vi "CAN.vi"() -> ()   [LabVIEW 2020]
uses:
  Global_Variable/Global.vi
  Global_Variable/A180648.vi
  Libraries/ZLG_CAN/ZLG_CAN.lvlib
panel:
  in  "CAN 通道":u32(ring) items=["0", "1"]
  in  "索引":u32(ring) items=["0", "1", "2", "3", "4", "5", "6", "7", "8"]
  in  "设备类型":u32(ring)=27 items=["PCI5121"=1, "PCI9810"=2, "USBCAN1"=3, "USBCAN2"=4, "PCI9820"=5, "PCI5110"=7, "PC104CAN"=11, "CANETUDP"=12, "PCI9840B"=14, "PC104C2"=15, "PCI9820I"=16, "CANETTCP"=17, "PCIE9221"=24, "PCI5010U"=19, "USBCAN_E_U"=20, "USBCAN_2E_U"=21, "PCI5020U"=22, "PCIE9120I"=27, "PCIE9110I"=28, "PCIE9140I"=29]
  in  "Stop":bool
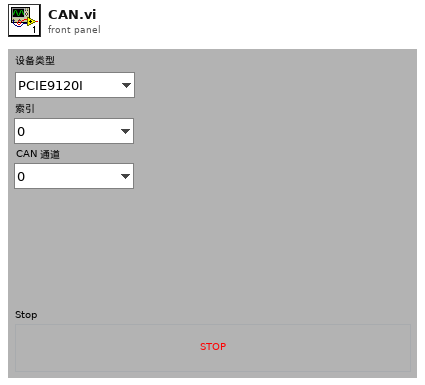
[diagram p1: front panel]
types:
  T1 = cluster{"波特率":u32, "ID":u32, "帧类型":enum8{"标准帧", "扩展帧"}, "帧格式":enum16{"数据帧", "远程帧"}, "周期(ms)":u32}
  T2 = typedef "ZLG_CAN.lvlib/Start_CAN (Reply Payload)--cluster.ctl" = cluster{"Success":bool, "Start_CAN_error":errorcluster}
  T3 = cluster{u8, u8, "y":u8, "y":u8, "y":u8, "y":u8, "y":u8, "y":u8}
  T4 = cluster{"y":u8, "y":u8, "y":u8, u8, u8, "y":u8, "y":u8, "y":u8}
  T5 = cluster{"[0]":u8, "[1]":u8, "[2]":u8, "[3]":u8, "[4]":u8, "[5]":u8, "[6]":u8, "[7]":u8}
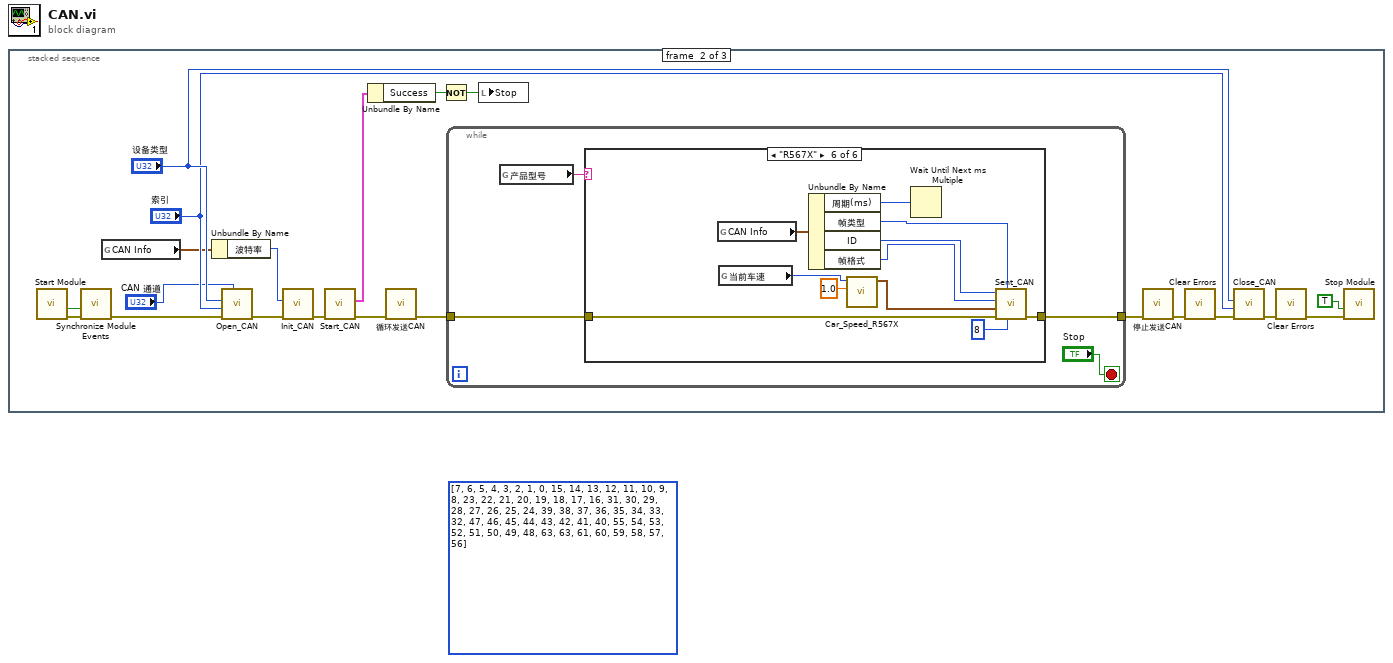
[diagram p0: block diagram]
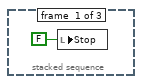
[diagram p2: hidden frame]
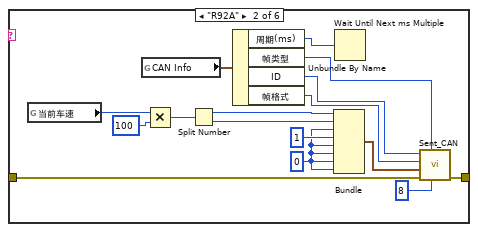
[diagram p4: hidden frame]
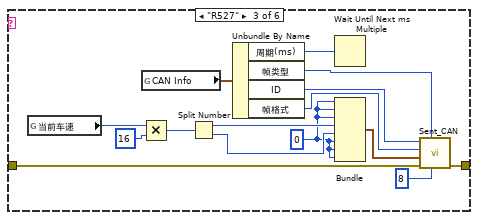
[diagram p5: hidden frame]
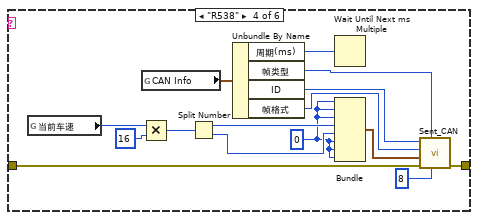
[diagram p6: hidden frame]
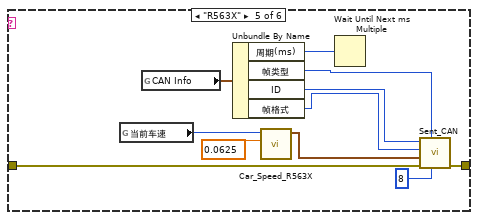
[diagram p7: hidden frame]
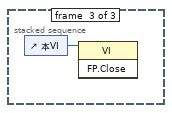
[diagram p8: hidden frame]
diagram:
  (unwired) i32[][] [[7, 6, 5, 4, 3, 2, 1, 0], [15, 14, 13, 12, 11, 10, 9, 8], [23, 22, 21, 20, 19, 18, 17, 16], [31, 30, 29, 28, 27, 26, 25, 24], [39, 38, 37, 36, 35, 34, 33, 32], [47, 46, 45, 44, 43, 42, 41, 40], [55, 54, 53, 52, 51, 50, 49, 48], [63, 63, 61, 60, 59, 58, 57, 56]]
  n1 = stacked-sequence {
    frame #0 {
      n2 = local write "Stop"(FALSE ("Stop")) -> ()
    }
    frame #1 {
      n3 = call "Start Module.vi"() -> ("error out"=w22:errorcluster, "Wait for Event Sync?"=w21:bool)  [unwired: 8 in, 2 out]
      n4 = call "Synchronize Module Events.vi"("error in (no error)"=w22, "Wait for Event Sync?"=w21) -> ("error out"=w20:errorcluster)  [unwired: 9 in]
      n5 = global read "Global.vi" "CAN Info"() -> (w7:T1)
      n6 = Unbundle By Name(w7) -> ("波特率"=w12:u32)
      n7 = call "Open_CAN.vi"("CAN 通道"="CAN 通道", "error in (no error)"=w20, "索引"="索引", "设备类型"="设备类型") -> ("error out"=w17:errorcluster)  [unwired: 7 in]
      n8 = call "Init_CAN.vi"("error in (no error)"=w17, "波特率"=w12) -> ("error out"=w13:errorcluster)  [unwired: 9 in]
      n9 = call "Start_CAN.vi"("error in (no error)"=w13) -> ("error out"=w6:errorcluster, "Reply Payload"=w15:T2)  [unwired: 8 in, 1 out]
      n10 = Unbundle By Name(w15) -> ("Success"=w14:bool)
      n11 = call "循环发送CAN.vi"("错误输入"=w6) -> ("错误输出"=w5:errorcluster)  [unwired: 10 in]
      n12 = Not(x=w14) -> (.not. x?=w2:bool)
      n13 = while {
        tunnel: w5 -> [w26]
        tunnel: [w25] -> w4
        stop <- "Stop" stop-if-true
        n14 = global read "Global.vi" "产品型号"() -> (w23:string)
        n15 = case shown="\"R567X\"" w23 {
          tunnel: w26 -> [w27 w43 w58 w73 w84 w95]
          tunnel: [w27 w42 w57 w72 w83 w94] -> w25
          frame "假", Default {
          }
          frame "R92A" {
            w28 = u8 0 ("y")
            n16 = global read "A180648.vi" "当前车速"() -> (w29:u16)
            n17 = global read "Global.vi" "CAN Info"() -> (w30:T1)
            n18 = Multiply(x=w29, y=u16 100) -> (x*y=w40:u16)
            n19 = Split Number(x=w40) -> (hi(x)=w39:u8, lo(x)=w38:u8)
            n20 = Unbundle By Name(w30) -> ("周期(ms)"=w34:u32, "帧类型"=w32:enum8{"标准帧", "扩展帧"}, "ID"=w31:u32, "帧格式"=w33:enum16{"数据帧", "远程帧"})
            n21 = Bundle(w39, w38, "y"=w28, "y"=u8 1, "y"=w28, "y"=w28, "y"=w28, "y"=w28) -> (w36:T3)  [unwired: 1 in]
            n22 = Wait Until Next ms Multiple(millisecond multiple=w34) -> ()  [unwired: 1 out]
            n23 = call "Sent_CAN.vi"("帧长度"=u8 8, "帧类型"=w32, "error in (no error)"=w43, "帧数据"=w36, "帧格式"=w33, "ID"=w31) -> ("error out"=w42:errorcluster)  [unwired: 5 in]
          }
          frame "R527" {
            w44 = u8 0 ("y")
            n24 = global read "A180648.vi" "当前车速"() -> (w47:u16)
            n25 = Multiply(x=w47, y=u16 16) -> (x*y=w55:u16)
            n26 = global read "Global.vi" "CAN Info"() -> (w48:T1)
            n27 = Split Number(x=w55) -> (hi(x)=w46:u8, lo(x)=w45:u8)
            n28 = Unbundle By Name(w48) -> ("周期(ms)"=w52:u32, "帧类型"=w50:enum8{"标准帧", "扩展帧"}, "ID"=w49:u32, "帧格式"=w51:enum16{"数据帧", "远程帧"})
            n29 = Wait Until Next ms Multiple(millisecond multiple=w52) -> ()  [unwired: 1 out]
            n30 = Bundle("y"=w44, "y"=w44, "y"=w44, w46, w45, "y"=w44, "y"=w44, "y"=w44) -> (w54:T4)  [unwired: 1 in]
            n31 = call "Sent_CAN.vi"("帧长度"=u8 8, "帧类型"=w50, "error in (no error)"=w58, "帧数据"=w54, "帧格式"=w51, "ID"=w49) -> ("error out"=w57:errorcluster)  [unwired: 5 in]
          }
          frame "R538" {
            w59 = u8 0 ("y")
            n32 = global read "A180648.vi" "当前车速"() -> (w62:u16)
            n33 = Multiply(x=w62, y=u16 16) -> (x*y=w70:u16)
            n34 = global read "Global.vi" "CAN Info"() -> (w63:T1)
            n35 = Split Number(x=w70) -> (hi(x)=w61:u8, lo(x)=w60:u8)
            n36 = Unbundle By Name(w63) -> ("周期(ms)"=w67:u32, "帧类型"=w65:enum8{"标准帧", "扩展帧"}, "ID"=w64:u32, "帧格式"=w66:enum16{"数据帧", "远程帧"})
            n37 = Wait Until Next ms Multiple(millisecond multiple=w67) -> ()  [unwired: 1 out]
            n38 = Bundle("y"=w59, "y"=w59, "y"=w59, w61, w60, "y"=w59, "y"=w59, "y"=w59) -> (w69:T4)  [unwired: 1 in]
            n39 = call "Sent_CAN.vi"("帧长度"=u8 8, "帧类型"=w65, "error in (no error)"=w73, "帧数据"=w69, "帧格式"=w66, "ID"=w64) -> ("error out"=w72:errorcluster)  [unwired: 5 in]
          }
          frame "R563X" {
            n40 = global read "A180648.vi" "当前车速"() -> (w75:u16)
            n41 = global read "Global.vi" "CAN Info"() -> (w77:T1)
            n42 = Unbundle By Name(w77) -> ("周期(ms)"=w81:u32, "帧类型"=w79:enum8{"标准帧", "扩展帧"}, "ID"=w78:u32, "帧格式"=w80:enum16{"数据帧", "远程帧"})
            n43 = call "Car_Speed_R563X.vi"("精度"=0.0625, "车速"=w75) -> ("报文"=w74:T5)  [unwired: 9 in]
            n44 = Wait Until Next ms Multiple(millisecond multiple=w81) -> ()  [unwired: 1 out]
            n45 = call "Sent_CAN.vi"("帧长度"=u8 8, "帧类型"=w79, "error in (no error)"=w84, "帧数据"=w74, "帧格式"=w80, "ID"=w78) -> ("error out"=w83:errorcluster)  [unwired: 5 in]
          }
          frame "R567X" {
            n46 = global read "Global.vi" "CAN Info"() -> (w88:T1)
            n47 = global read "A180648.vi" "当前车速"() -> (w86:u16)
            n48 = Unbundle By Name(w88) -> ("周期(ms)"=w92:u32, "帧类型"=w90:enum8{"标准帧", "扩展帧"}, "ID"=w89:u32, "帧格式"=w91:enum16{"数据帧", "远程帧"})
            n49 = call "Car_Speed_R567X.vi"("精度"=1.0, "车速"=w86) -> ("报文"=w87:T5)  [unwired: 9 in]
            n50 = Wait Until Next ms Multiple(millisecond multiple=w92) -> ()  [unwired: 1 out]
            n51 = call "Sent_CAN.vi"("帧长度"=u8 8, "帧类型"=w90, "error in (no error)"=w95, "帧数据"=w87, "帧格式"=w91, "ID"=w89) -> ("error out"=w94:errorcluster)  [unwired: 5 in]
          }
        }
      }
      n52 = local write "Stop"(w2) -> ()
      n53 = call "停止发送CAN.vi"("错误输入"=w4) -> ("错误输出"=w3:errorcluster)  [unwired: 10 in]
      n54 = call <vilib>:"Clear Errors.vi"("error in (no error)"=w3) -> ("error out"=w8:errorcluster)  [unwired: 5 in, 1 out]
      n55 = call "Close_CAN.vi"("error in (no error)"=w8, "索引"="索引", "设备类型"="设备类型") -> ("error out"=w11:errorcluster)  [unwired: 8 in]
      n56 = call <vilib>:"Clear Errors.vi"("error in (no error)"=w11) -> ("error out"=w9:errorcluster)  [unwired: 5 in, 1 out]
      n57 = call "Stop Module.vi"("error in (no error)"=w9, "Wait for Module to Stop? (F)"=TRUE) -> ()  [unwired: 9 in, 1 out]
    }
    frame #2 {
      n58 = control-ref of="本VI"() -> (w96:refnum<vi>)
      n59 = invoke class="VI" method="FP.Close"(reference=w96) -> ()  [unwired: 2 in, 3 out]
    }
  }
